vi "shooterBangBang.vi"(10 "CounterDevRef in":T1, 11 "rpmTarget":dbl) -> (3 "Output":dbl)   [LabVIEW 2012]
uses:
  <vilib>/Rock Robotics/WPI/Counter/WPI_CounterDevRef.ctl
  <vilib>/Rock Robotics/SystemInterfaces/Counter/FPGA_CounterCtrSystemIndex.ctl
panel:
  out "withinMotorRange":bool
  in  "rpmRange":dbl
  out "rpmCurrent":dbl
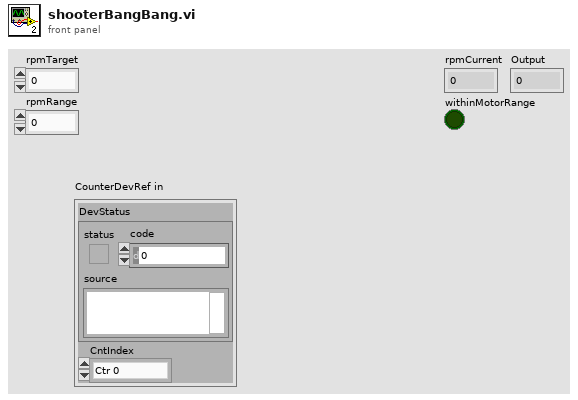
[diagram p1: front panel]
types:
  T1 = typedef "WPI_CounterDevRef.ctl" = cluster{"DevStatus":errorcluster, "CntIndex":T2}
  T2 = typedef "FPGA_CounterCtrSystemIndex.ctl" = enum8{"Ctr 0", "Ctr 1", "Ctr 2", "Ctr 3", "Ctr 4", "Ctr 5", "Ctr 6", "Ctr 7", "Invalid"}
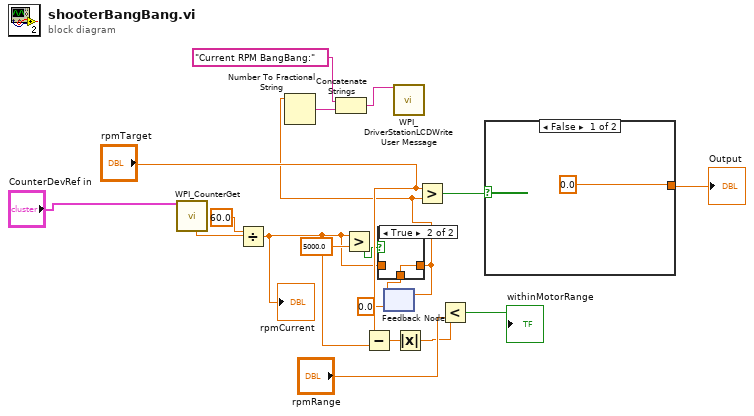
[diagram p0: block diagram]
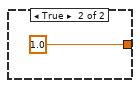
[diagram p3: hidden frame]
diagram:
  n1 = call <vilib>:"WPI_CounterGet.vi"("CounterDevRef in"="CounterDevRef in") -> ("Period (sec)"=w19:dbl)  [unwired: 5 in, 5 out]
  n2 = Divide(x=60.0, y=w19) -> (x/y=w4:dbl)
  "rpmCurrent" <- w4
  n3 = Greater?(x=w4, y=5000.0) -> (0:w5:bool)
  n4 = Subtract(x="rpmTarget", y=w4) -> (x-y=w14:dbl)
  n5 = feedback #1(0.0) -> (w2:dbl)
  n6 = case shown="True" w5 {
    tunnel: w4 -> [w20 _]
    tunnel: [w20 w21] -> w3
    tunnel: w2 -> [_ w21]
    frame False {
    }
    frame True {
    }
  }
  n7 = Number To Fractional String(number=w3) -> (F-format string=w9:string)  [unwired: 3 in]
  n8 = Concatenate Strings("Current RPM BangBang:" ("string"), w9) -> (w7:string)
  n9 = feedback-in #1(w3) -> ()
  n10 = call <vilib>:"WPI_DriverStationLCDWrite User Message.vi"("line text"=w7) -> ()  [unwired: 14 in, 1 out]
  n11 = Absolute Value(x=w14) -> (abs(x)=w13:dbl)
  n12 = Greater?(x="rpmTarget", y=w3) -> (0:w17:bool)
  n13 = Less?(x=w13, y="rpmRange") -> (x < y?=→"withinMotorRange":bool)
  n14 = case shown="False" w17 {
    tunnel: [0.0 ("Output") 1.0 ("Output")] -> w16
    frame False {
    }
    frame True {
    }
  }
  "Output" <- w16
